vi "_PluginLoader_StopPlugins.vi"(8 "error in (no error)":errorcluster, 11 "_PluginLoader in":refnum<class "_PluginLoader.lvclass">) -> (0 "error out":errorcluster, 3 "_PluginLoader out":refnum<class "_PluginLoader.lvclass">)   [LabVIEW 2014, in "_PluginLoader.lvclass"]
uses:
  _PluginLoader.lvclass
  _PluginLoader.lvclass/_PluginLoader.ctl
  GCMPlugin/GCMPlugin.lvclass
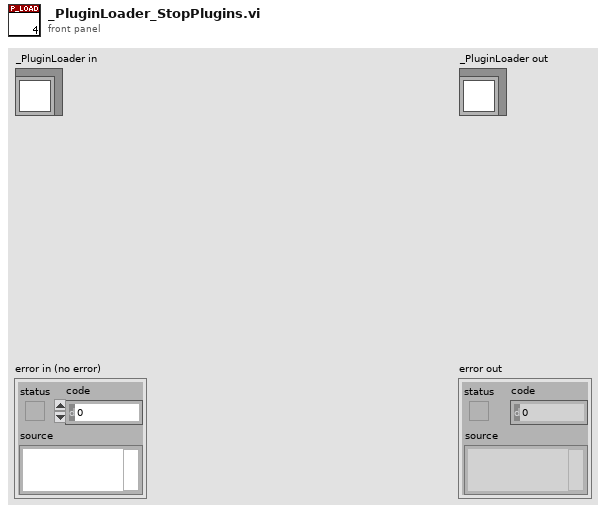
[diagram p1: front panel]
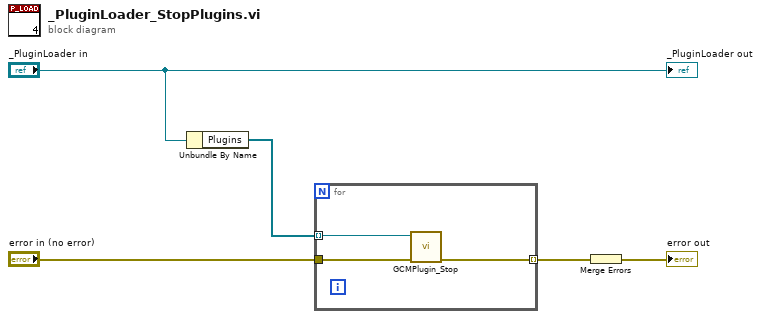
[diagram p0: block diagram]
diagram:
  n1 = Unbundle By Name("_PluginLoader in") -> ("Plugins"=w2:refnum<class "GCMPlugin.lvclass">[])
  n2 = for {
    tunnel: w2 -> [w8] mode=indexing
    tunnel: [w7] -> w1 mode=indexing
    tunnel: "error in (no error)" -> [w6]
    n3 = call "GCMPlugin_Stop.vi"("error in (no error)"=w6, "_LVCMPlugin in"=w8) -> ("error out"=w7:errorcluster)  [unwired: 8 in, 1 out]
  }
  n4 = Merge Errors(w1) -> (→"error out":errorcluster)
  "_PluginLoader out" <- "_PluginLoader in"
